vi "ContinuosSplitMicroSettings.vi"(0 "Loop Microscope Settings":string[][](array[string])) -> (4 "Microscope":T1(array[cluster]))   [LabVIEW 2018, in "ContinousLoop.lvlib"]
uses:
  ContinousLoop.lvlib
panel:
  out "Exposure Time":i32[](array[numeric])
  out "Intensity":dbl[](array[numeric])
  out "Prism":string[](array[string])
  out "Filter":string[](array[string])
  out "Objective":i32[](array[numeric])
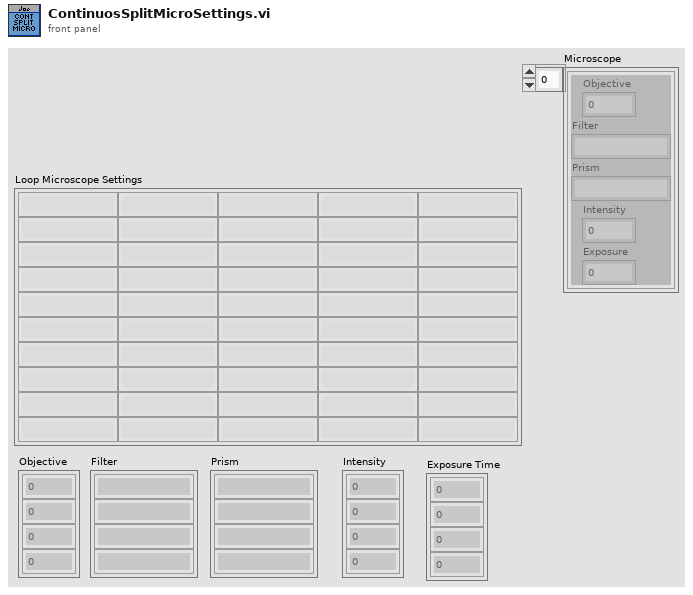
[diagram p1: front panel]
types:
  T1 = cluster{"Objective":i32, "Filter":string, "Prism":string, "Intensity":dbl, "Exposure":i32}[]
  T2 = cluster{"Objective":i32, "Filter":string, "Prism":string, "Intensity":dbl, "Exposure":i32}
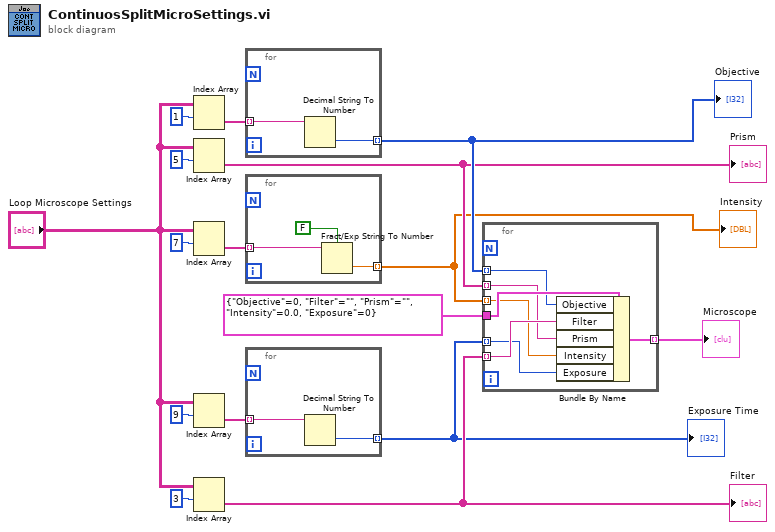
[diagram p0: block diagram]
diagram:
  n1 = Index Array(array="Loop Microscope Settings", index (row)=1) -> (element=w15:string[])  [unwired: 1 in]
  n2 = Index Array(array="Loop Microscope Settings", index (row)=5) -> (element=w4:string[])  [unwired: 1 in]
  "Prism" <- w4
  n3 = Index Array(array="Loop Microscope Settings", index (row)=7) -> (element=w8:string[])  [unwired: 1 in]
  n4 = Index Array(array="Loop Microscope Settings", index (row)=9) -> (element=w9:string[])  [unwired: 1 in]
  n5 = Index Array(array="Loop Microscope Settings", index (row)=3) -> (element=w5:string[])  [unwired: 1 in]
  "Filter" <- w5
  n6 = for {
    tunnel: w15 -> [w18] mode=indexing
    tunnel: [w17] -> w6 mode=indexing
    n7 = Decimal String To Number(string=w18) -> (number=w17:i32)  [unwired: 2 in, 1 out]
  }
  "Objective" <- w6
  n8 = for {
    tunnel: w8 -> [w21] mode=indexing
    tunnel: [w20] -> w3 mode=indexing
    n9 = Fract/Exp String To Number(use system decimal point (T)=FALSE, string=w21) -> (number=w20:dbl)  [unwired: 2 in, 1 out]
  }
  "Intensity" <- w3
  n10 = for {
    tunnel: w9 -> [w23] mode=indexing
    tunnel: [w22] -> w2 mode=indexing
    n11 = Decimal String To Number(string=w23) -> (number=w22:i32)  [unwired: 2 in, 1 out]
  }
  "Exposure Time" <- w2
  n12 = for {
    tunnel: T2 {"Objective"=0, "Filter"="", "Prism"="", "Intensity"=0.0, "Exposure"=0} -> [w30]
    tunnel: w6 -> [w29] mode=indexing
    tunnel: w5 -> [w28] mode=indexing
    tunnel: w4 -> [w27] mode=indexing
    tunnel: w3 -> [w26] mode=indexing
    tunnel: w2 -> [w25] mode=indexing
    tunnel: [w24] -> w1 mode=indexing
    n13 = Bundle By Name(cluster=w30, "Objective"=w29, "Filter"=w28, "Prism"=w27, "Intensity"=w26, "Exposure"=w25) -> (w24:T2)
  }
  "Microscope" <- w1
